vi "XLP80_EA_Select Device.vi"(6 "EA Type":enum16{"Batterie", "Stack", "Rekuperation"}(ring), 8 "err in":errorcluster) -> (0 "err out":errorcluster, 3 "Device information":string[](array[string]))   [LabVIEW 2021]
panel:
  out "Device array":T1(array[cluster])
  out "Device information array":string[][](array[string])
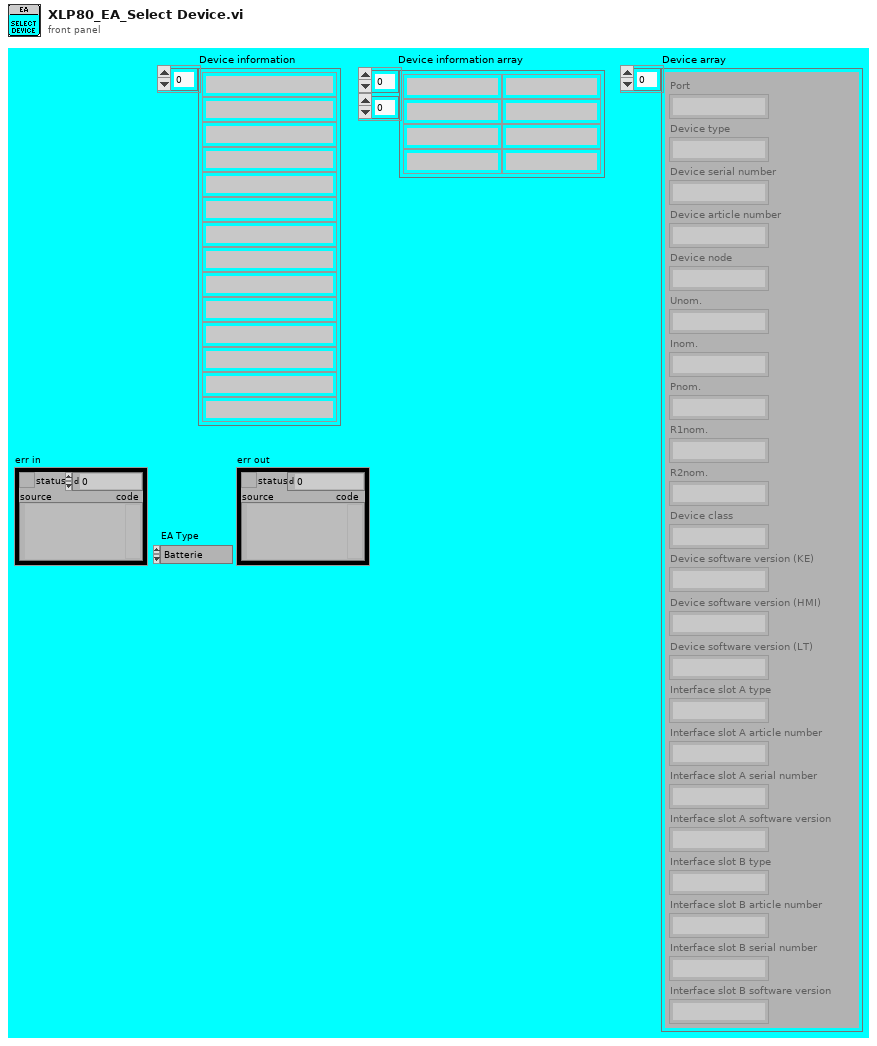
[diagram p1: front panel]
types:
  T1 = cluster{"Port":string, "Device type":string, "Device serial number":string, "Device article number":string, "Device node":string, "Unom.":string, "Inom.":string, "Pnom.":string, "R1nom.":string, "R2nom.":string, "Device class":string, "Device software version (KE)":string, "Interface slot A type":string, "Interface slot A article number":string, "Interface slot A serial number":string, "Interface slot A software version":string, "Interface slot B type":string, "Interface slot B article number":string, "Interface slot B serial number":string, "Interface slot B software version":string, "Device software version (HMI)":string, "Device software version (LT)":string}[]
  T2 = cluster{"IP range start":u8[], "IP range end":u8[], "Port":u16}
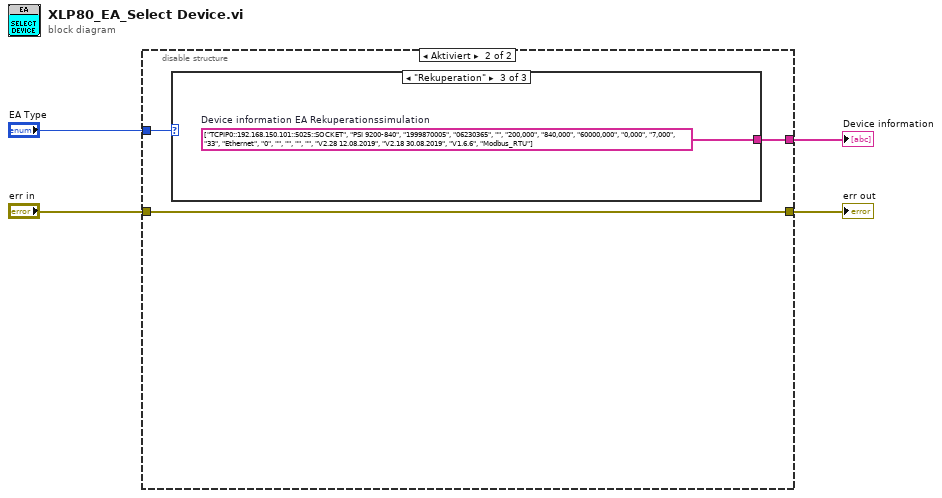
[diagram p0: block diagram]
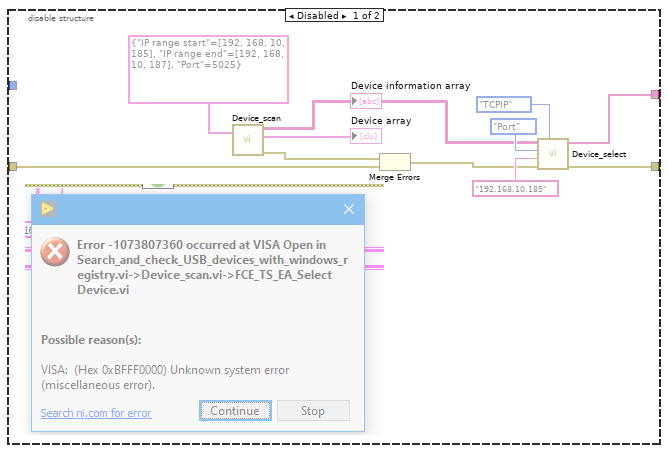
[diagram p2: hidden frame]
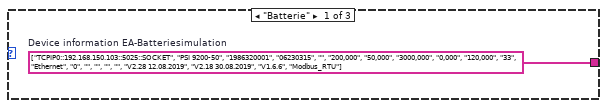
[diagram p3: hidden frame]
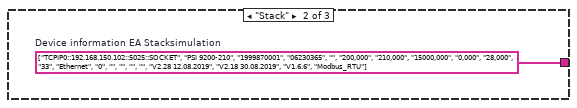
[diagram p4: hidden frame]
diagram:
  n1 = disable-structure shown="Aktiviert" {
    disable-tunnel: [w13 w18] -> w4
    disable-tunnel: [w12 w16] -> w3
    disable-tunnel: "err in" -> [w7 w18]
    disable-tunnel: "EA Type" -> [_ w17]
    frame Disabled {
      n2 = call <instrlib>:"Device_scan.vi"("IP settings"=T2 {"IP range start"=[192, 168, 10, 185], "IP range end"=[192, 168, 10, 187], "Port"=5025}) -> ("Device information array"=w5:string[][], "Device array"=→"Device array":T1, "error out"=w10:errorcluster)  [unwired: 1 in, 1 out]
      "Device information array" <- w5
      n3 = Merge Errors(w10, w7) -> (w8:errorcluster)
      n4 = call <instrlib>:"Device_select.vi"("Reference"=enum16{"ASRL/COM", "GPIB", "TCPIP"}."TCPIP", "error in (no error)"=w8, "Alias"="192.168.10.185" ("Number/Alias"), "Open by"=enum16{"Device Node", "Serial number", "Port"}."Port", "Device information array"=w5) -> ("error out"=w13:errorcluster, "Device information"=w12:string[])  [unwired: 2 in]
    }
    frame Enabled {
      n5 = case shown="\"Rekuperation\"" w17 {
        tunnel: [w19 w20 w21] -> w16
        frame "Batterie" {
          w19 = string[] ["TCPIP0::192.168.150.103::5025::SOCKET", "PSI 9200-50", "1986320001", "06230315", "", "200,000", "50,000", "3000,000", "0,000", "120,000", "33", "Ethernet", "0", "", "", "", "", "V2.28 12.08.2019", "V2.18 30.08.2019", "V1.6.6", "Modbus_RTU"]  # Device information EA-Batteriesimulation
        }
        frame "Stack" {
          w20 = string[] ["TCPIP0::192.168.150.102::5025::SOCKET", "PSI 9200-210", "1999870001", "06230365", "", "200,000", "210,000", "15000,000", "0,000", "28,000", "33", "Ethernet", "0", "", "", "", "", "V2.28 12.08.2019", "V2.18 30.08.2019", "V1.6.6", "Modbus_RTU"]  # Device information EA Stacksimulation
        }
        frame "Rekuperation" {
          w21 = string[] ["TCPIP0::192.168.150.101::5025::SOCKET", "PSI 9200-840", "1999870005", "06230365", "", "200,000", "840,000", "60000,000", "0,000", "7,000", "33", "Ethernet", "0", "", "", "", "", "V2.28 12.08.2019", "V2.18 30.08.2019", "V1.6.6", "Modbus_RTU"]  # Device information EA Rekuperationssimulation
        }
      }
    }
  }
  "err out" <- w4
  "Device information" <- w3
